vi "SubtractMeanFromPoints.vi"(8 "error in":errorcluster, 11 "x":T1) -> (0 "error out":errorcluster, 1 "var(x)":dbl format="%0.2f", 2 "mean(x)":dbl[](array[numeric]), 3 "x - mean(x)":dbl[][](array[numeric]))   [LabVIEW 2020, in "ar.lvlib"]
uses:
  ar.lvlib
  PointSet.ctl
  <vilib>/Analysis/baseanly.llb/Mean (DBL).vi
  <vilib>/ErrorRing/Error Ring.xnode
  <vilib>/Analysis/NI_AALBase.lvlib
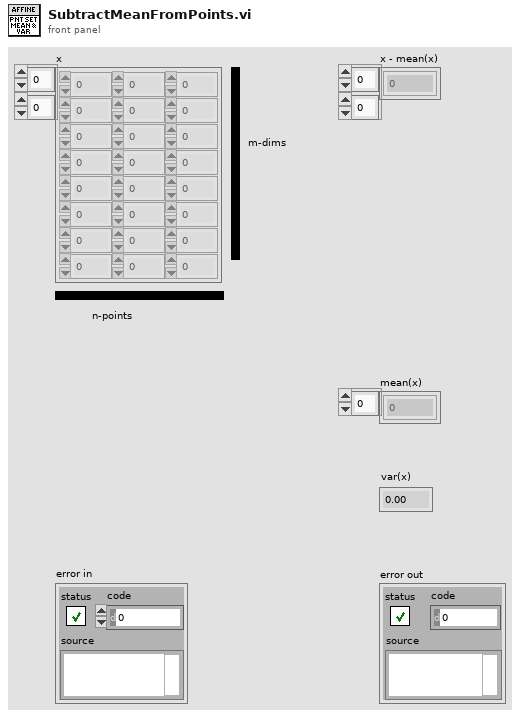
[diagram p1: front panel]
types:
  T1 = typedef "ar.lvlib/PointSet.ctl" = dbl[][]
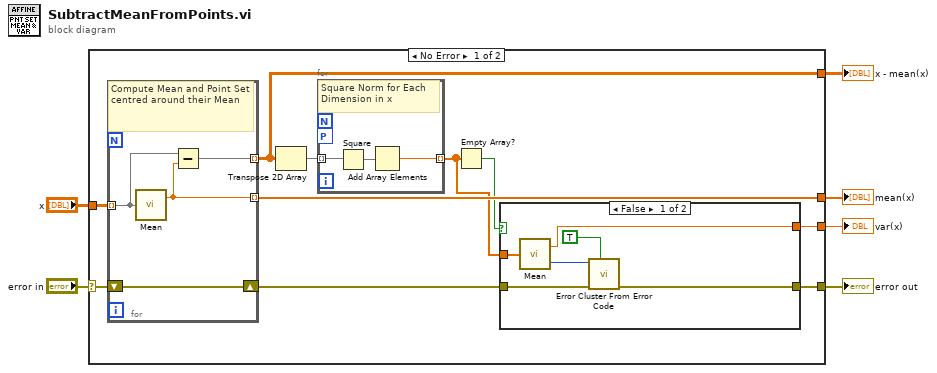
[diagram p0: block diagram]
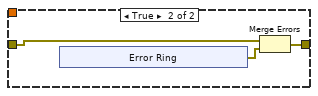
[diagram p2: hidden frame]
diagram:
  n1 = case shown="No Error" "error in" {
    selector: "error in" -> [w11 w38]
    tunnel: [w16 _] -> w6
    tunnel: "x" -> [w15 _]
    tunnel: [w13 _] -> w4
    tunnel: [w12 _] -> w3
    tunnel: [w9 w38] -> w1
    frame No Error {
      n2 = for {
        tunnel: w15 -> [w37] mode=indexing
        tunnel: [w36] -> w16 mode=indexing
        tunnel: [w35] -> w13 mode=indexing
        shift-right: [w34] -> w10
        shift-left: w11 -> [w34]
        # "Compute Mean and Point Set centred around their Mean"
        n3 = call-poly <vilib>:"Mean.vi"("X"=w37) -> ("mean"=w36:dbl)  [unwired: 1 out]
        n4 = Subtract(x=w37, y=w36) -> (x-y=w35:dbl[])
      }
      n5 = Transpose 2D Array(2D array=w13) -> (transposed array=w14:dbl[][])
      n6 = for {
        tunnel: w14 -> [w33] mode=indexing
        tunnel: [w31] -> w8 mode=indexing
        workers-P: _ -> [_]
        # "Square Norm for Each Dimension in x"
        n7 = Square(x=w33) -> (x^2=w32:dbl[])
        n8 = Add Array Elements(numeric array=w32) -> (sum=w31:dbl)
      }
      n9 = Empty Array?(array=w8) -> (empty?=w7:bool)
      n10 = case shown="False" w7 {
        tunnel: [w22 _] -> w12
        tunnel: w10 -> [w20 w25]
        tunnel: [w19 w24] -> w9
        tunnel: w8 -> [w18 _]
        frame False {
          n11 = call-poly <vilib>:"Mean.vi"("X"=w18) -> ("mean"=w22:dbl, "error"=w21:i32)
          n12 = call <vilib>:"Error Cluster From Error Code.vi"("show call chain? (False)"=TRUE, "error in (no error)"=w20, "error code (0)"=w21) -> ("error out"=w19:errorcluster)  [unwired: 6 in]
        }
        frame True {
          n13 = xnode "Error Ring"() -> ("error out"=w23:errorcluster)
          n14 = Merge Errors(w25, w23) -> (w24:errorcluster)
        }
      }
    }
    frame Error {
    }
  }
  "x - mean(x)" <- w4
  "mean(x)" <- w6
  "var(x)" <- w3
  "error out" <- w1
